vi "Calculate Metrics.vi"(0 "Application In":refnum<class "Application.lvclass">, 5 "Input Values":T3, 7 "Error Percentage":dbl, 9 "INL Method":T1=enum."End Point", 11 "Error In":errorcluster) -> (2 "Monotonic?":bool, 4 "Application Out":refnum<class "Application.lvclass">, 6 "DNL Values":dbl[](array[numeric]), 8 "INL Values":dbl[](array[numeric]), 10 "Transfer Function":T2, 15 "Error Out":errorcluster)   [LabVIEW 2023, in "Application.lvclass"]
doc: "The VI acts as a API to calculate all the metrics required for INL and DNL testing."
uses:
  Application.lvclass
  Typedef/Input Voltage Parameters.ctl
  Typedef/Transfer Function.ctl
  Typedef/INL Method.ctl
  Mode/Mode.lvclass
  C:/Users/Ancy.Augustin/Downloads/Tasks (2)/Tasks/Tasks/SDLC - DNL and INL Testing/SDLC - DNL and INL Testing/INL and DNL Calculation/Classes/Application/Application.lvclass
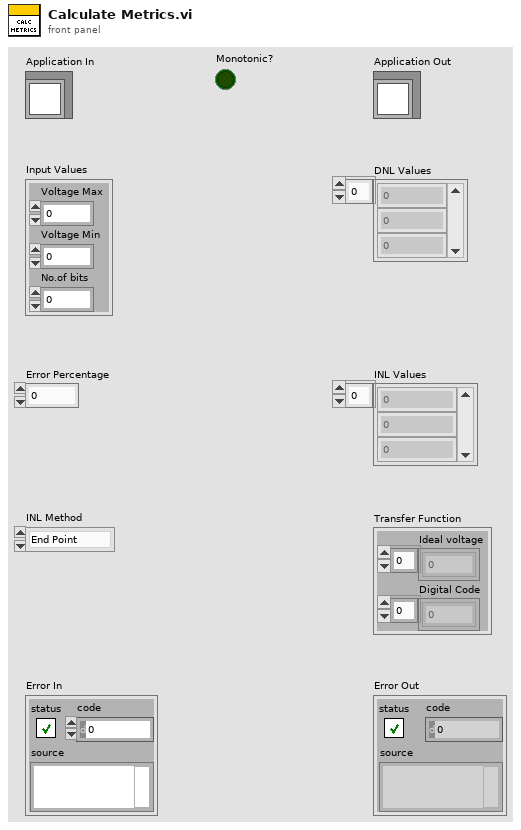
[diagram p1: front panel]
types:
  T1 = typedef "INL Method.ctl" = enum16{"Best Fit", "End Point"}
  T2 = typedef "Transfer Function.ctl" = cluster{"Ideal voltage":dbl[], "Digital Code":dbl[]}
  T3 = typedef "Input Voltage Parameters.ctl" = cluster{"Voltage Max":dbl, "Voltage Min":dbl, "No.of bits":dbl}
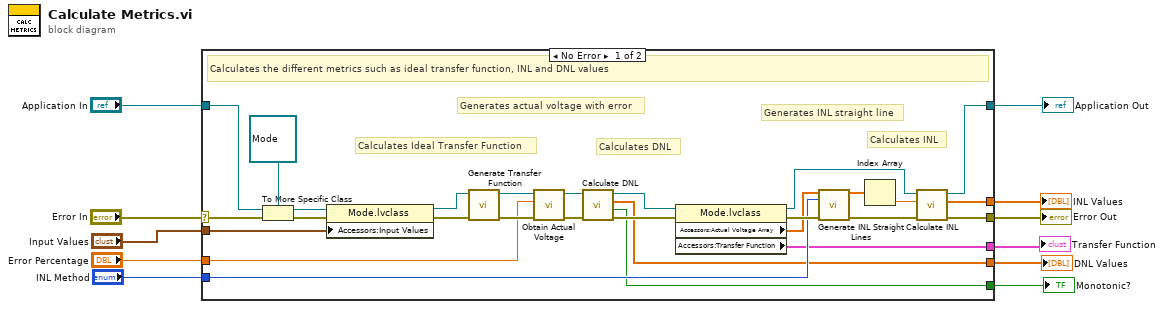
[diagram p0: block diagram]
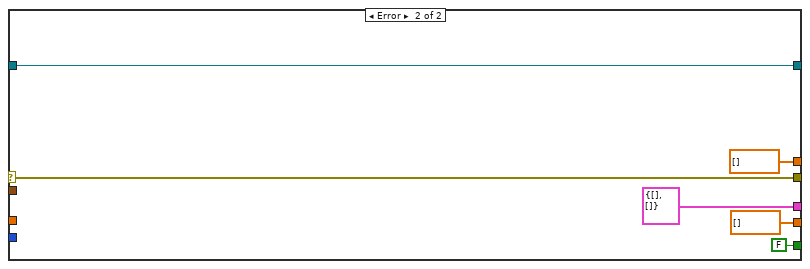
[diagram p2: hidden frame]
diagram:
  n1 = case shown="No Error" "Error In" {
    selector: "Error In" -> [w39 w45]
    tunnel: [w20 w45] -> w10
    tunnel: "Input Values" -> [w32 _]
    tunnel: [w15 dbl[] [] ("DNL")] -> w8
    tunnel: [w14 dbl[] [] ("INL")] -> w7
    tunnel: "INL Method" -> [w21 _]
    tunnel: "Application In" -> [w36 w41]
    tunnel: "Error Percentage" -> [w28 _]
    tunnel: [w16 T2 {"Ideal voltage"=[], "Digital Code"=[]} ("Accessors:Transfer Function")] -> w3
    tunnel: [w13 w41] -> w2
    tunnel: [w12 FALSE ("Monotonic?")] -> w1
    frame No Error {
      # "Calculates INL"
      # "Generates INL straight line"
      # "Calculates DNL"
      # "Generates actual voltage with error"
      # "Calculates Ideal Transfer Function"
      # "Calculates the different metrics such as ideal transfer function, INL and DNL values"
      n2 = To More Specific Class(target class=refnum<class "Mode.lvclass"> refnum ("Mode.lvclass"), reference=w36, error in=w39) -> (specific class reference=w33:refnum<class "Mode.lvclass">, error out=w37:errorcluster)
      n3 = property class="Mode.lvclass"(reference=w33, error in=w37, "Accessors:Input Values"=w32) -> (reference out=w31:refnum<class "Mode.lvclass">, error out=w34:errorcluster)
      n4 = call-dynamic "Generate Transfer Function.vi"("Error In"=w34, "Mode In"=w31) -> ("Error Out"=w38:errorcluster, "Mode Out"=w29:refnum<class "Mode.lvclass">)  [unwired: 8 in]
      n5 = call-dynamic "Obtain Actual Voltage.vi"("Error In"=w38, "Error Percentage"=w28, "Mode in"=w29) -> ("Error Out"=w30:errorcluster, "Mode out"=w25:refnum<class "Mode.lvclass">)  [unwired: 7 in]
      n6 = call-dynamic "Calculate DNL.vi"("Error In"=w30, "Mode in"=w25) -> ("Error Out"=w27:errorcluster, "Monotonic?"=w12:bool, "DNL"=w15:dbl[], "Mode out"=w23:refnum<class "Mode.lvclass">)  [unwired: 6 in]
      n7 = property class="Mode.lvclass"(reference=w23, error in=w27) -> (reference out=w18:refnum<class "Mode.lvclass">, error out=w24:errorcluster, "Accessors:Actual Voltage Array"=w22:dbl[], "Accessors:Transfer Function"=w16:T2)
      n8 = call "Generate INL Straight Lines.vi"("Actual voltage array"=w22, "INL Method"=w21, "Error In"=w24) -> ("Straight Line"=w19:dbl[], "Error Out"=w26:errorcluster)  [unwired: 11 in]
      n9 = Index Array(array=w19) -> (element=w17:dbl)  [unwired: 1 in]
      n10 = call-dynamic "Calculate INL.vi"("Error In"=w26, "V Zero"=w17, "Mode in"=w18) -> ("Error Out"=w20:errorcluster, "INL"=w14:dbl[], "Mode out"=w13:refnum<class "Mode.lvclass">)  [unwired: 6 in]
    }
    frame Error {
    }
  }
  "Error Out" <- w10
  "Transfer Function" <- w3
  "DNL Values" <- w8
  "INL Values" <- w7
  "Application Out" <- w2
  "Monotonic?" <- w1
